vi "filters_to_xml.vi"(8 "error in":errorcluster, 11 "Filter Settings":T1) -> (0 "error out":errorcluster, 3 "filter settings string":string)   [LabVIEW 2013]
doc: "Saves filter settings to xml in the format:\n\n<CounterFilterMinimum>\n<bin>%u\\t</bin>\n</CounterFilterMinimum>\n<ROIFiltersMinimum>\n<shot>%u\\t</shot>\n</ROIFiltersMinimum>\n\nMTL 2013 Jan 1"
uses:
  filters.ctl
panel:
  # "Regions of Interest -->"
  # "Shots\n   |\n  V"
  # "Counters -->"
  # "Counter\n    bins\n       |\n      V"
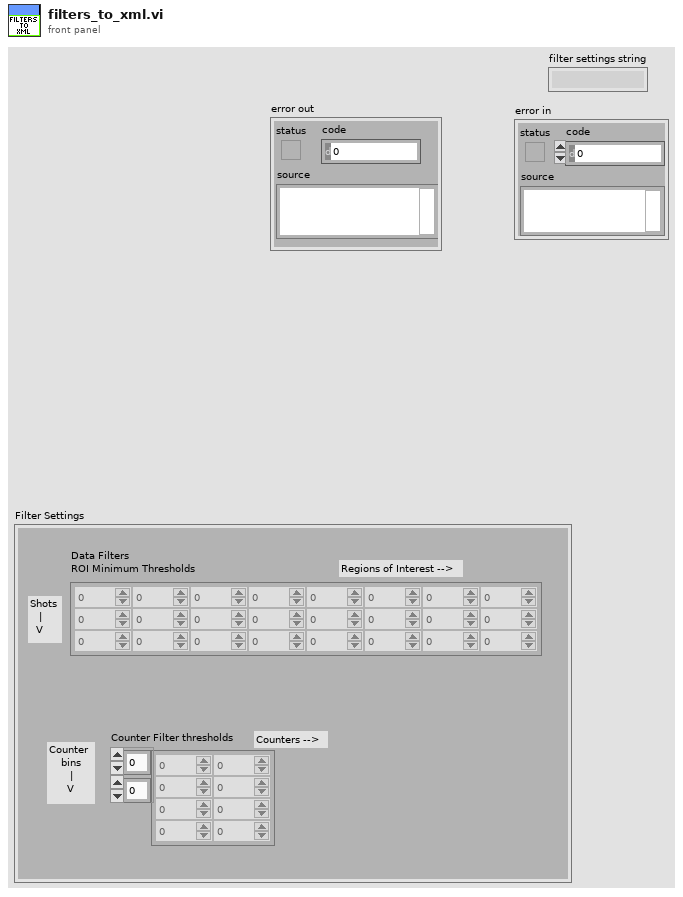
[diagram p1: front panel]
types:
  T1 = typedef "filters.ctl" = cluster{"Counter Filter thresholds":u32[][], "Data Filters\nROI Minimum Thresholds":u64[][]}
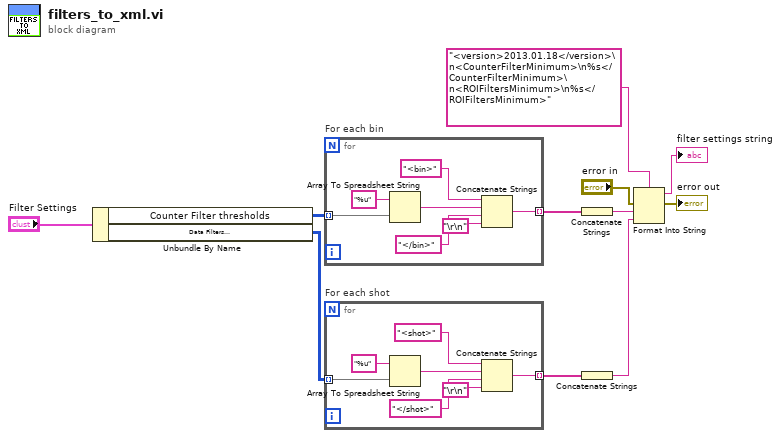
[diagram p0: block diagram]
diagram:
  n1 = Unbundle By Name("Filter Settings") -> ("Counter Filter thresholds"=w7:u32[][], "Data Filters\nROI Minimum Thresholds"=w4:u64[][])
  n2 = for "For each bin" {
    tunnel: w7 -> [w17] mode=indexing
    tunnel: [w12] -> w6 mode=indexing
    n3 = Array To Spreadsheet String(array=w17, 3:"%u" ("format string")) -> (spreadsheet string=w16:string)  [unwired: 1 in]
    n4 = Concatenate Strings("<bin>" ("string"), w16, "</bin>" ("string"), "\r\n") -> (w12:string)
  }
  n5 = for "For each shot" {
    tunnel: w4 -> [w24] mode=indexing
    tunnel: [w19] -> w3 mode=indexing
    n6 = Array To Spreadsheet String(array=w24, 3:"%u" ("format string")) -> (spreadsheet string=w23:string)  [unwired: 1 in]
    n7 = Concatenate Strings("<shot>" ("string"), w23, "</shot>" ("string"), "\r\n") -> (w19:string)
  }
  n8 = Concatenate Strings(w6) -> (w5:string)
  n9 = Concatenate Strings(w3) -> (w2:string)
  n10 = Format Into String(format string="<version>2013.01.18</version>\n<CounterFilterMinimum>\n%s</CounterFilterMinimum>\n<ROIFiltersMinimum>\n%s</ROIFiltersMinimum>", error in="error in", w5, w2) -> (resulting string=→"filter settings string":string, error out=→"error out":errorcluster)  [unwired: 1 in]
